vi "Untitled 1.vi"() -> ()   [LabVIEW 2023]
uses:
  <vilib>/DAQmx/read.llb/DAQmx Read (Analog 1D Wfm NChan NSamp).vi
  <vilib>/measure/NI_MAPro.lvlib
  <vilib>/measure/matone.llb/Extract Single Tone Information N Chan.vi
  <vilib>/Analysis/NI_AALPro.lvlib
panel:
  out "Settle Time":dbl
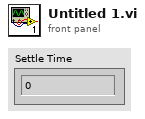
[diagram p1: front panel]
types:
  T1 = cluster{"slope min":dbl, "slope max":dbl, "intercept min":dbl, "intercept max":dbl}
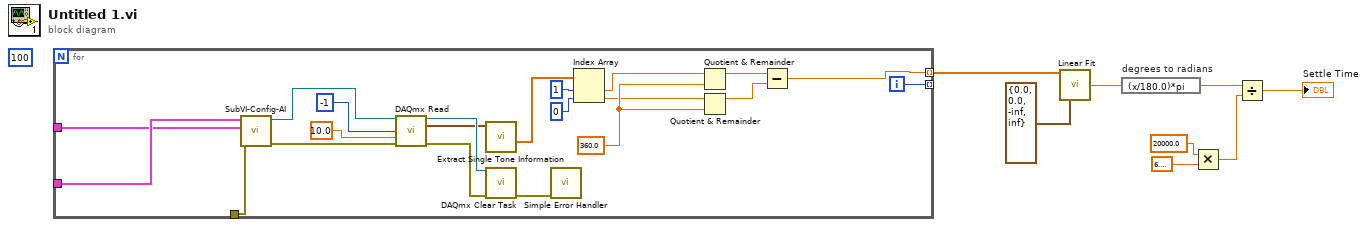
[diagram p0: block diagram]
diagram:
  (unwired) 100
  n1 = for {
    tunnel: _ -> [w24]
    tunnel: _ -> [w23]
    tunnel: [w19] -> w8 mode=indexing
    tunnel: [w16] -> _ mode=indexing
    tunnel: _ -> [w10]
    i -> [w16]
    w15 = 360.0 ("y")
    n2 = call "SubVI-Config-AI.vi"("error in (no error)"=w10, "Channels"=w23, "Timing Params"=w24) -> ("error out"=w26:errorcluster, "Refnum out"=w29:refnum<k21>)  [unwired: 7 in]
    n3 = call-poly <vilib>:"DAQmx Read.vi"("task/channels in"=w29, "number of samples per channel"=-1, "timeout"=10.0, "error in"=w26) -> ("task out"=w28:refnum<k21>, "data"=w18:waveform(dbl)[], "error out"=w27:errorcluster)  [unwired: 9 in]
    n4 = call-poly <vilib>:"Extract Single Tone Information.vi"("time signals in"=w18) -> ("detected phases (deg)"=w17:dbl[])  [unwired: 5 in, 5 out]
    n5 = call <vilib>:"DAQmx Clear Task.vi"("task in"=w28, "error in"=w27) -> ("error out"=w22:errorcluster)  [unwired: 13 in]
    n6 = call <vilib>:"Simple Error Handler.vi"("error in (no error)"=w22) -> ()  [unwired: 4 in, 5 out]
    n7 = Index Array(array=w17, index #1=1 ("index"), index #2=0 ("index")) -> (element #1=w14:dbl, element #2=w13:dbl)
    n8 = Quotient & Remainder(x=w14, y=w15) -> (x-y*floor(x/y)=w12:dbl)  [unwired: 1 out]
    n9 = Quotient & Remainder(x=w13, y=w15) -> (x-y*floor(x/y)=w11:dbl)  [unwired: 1 out]
    n10 = Subtract(x=w12, y=w11) -> (x-y=w19:dbl)
  }
  n11 = call <vilib>:"Linear Fit.vi"("Y"=w8, "parameter bounds"=T1 {"slope min"=0.0, "slope max"=0.0, "intercept min"=-inf, "intercept max"=inf}) -> ("X"=w7:dbl[], "intercept"=w6:dbl)  [unwired: 8 in, 4 out]
  n12 = expression code="(x/180.0)*pi" "degrees to radians"(w6) -> (w2:dbl)
  n13 = Multiply(x=20000.0, y=6.283185307179586) -> (x*y=w3:dbl)
  n14 = Divide(x=w2, y=w3) -> (x/y=→"Settle Time":dbl)
